vi "ws Spartan Event Log.vi"(4 "Force Archive? (f)":bool, 5 "error in (no error)":errorcluster, 6 "username (\"\")":string, 7 "module (\"\")":string, 8 "message (\"\")":string) -> (0 "error out":errorcluster)   [LabVIEW 2011]
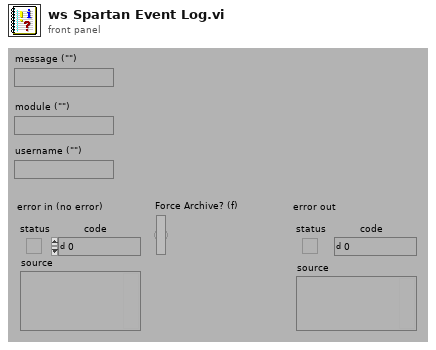
[diagram p1: front panel]
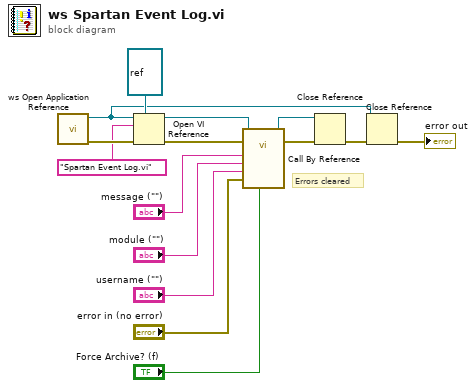
[diagram p0: block diagram]
diagram:
  # "Errors cleared"
  n1 = call "ws Open Application Reference.vi"() -> ("error out"=w15:errorcluster, "application reference"=w2:refnum<vi>)  [unwired: 10 in]
  n2 = Open VI Reference(type specifier VI Refnum (for type only)=refnum<vi> refnum, application reference (local)=w2, vi path="Spartan Event Log.vi", error in (no error)=w15) -> (vi reference=w11:refnum<vi>, error out=w13:errorcluster)  [unwired: 2 in]
  n3 = call-by-ref "?"(reference=w11, error in=w13, "Force Archive? (f)"="Force Archive? (f)", 5:"error in (no error)"="error in (no error)", "username (\"\")"="username (\"\")", "module (\"\")"="module (\"\")", "message (\"\")"="message (\"\")") -> (reference out=w5:refnum<vi>, error out=w4:errorcluster)  [unwired: 3 in, 1 out]
  n4 = Close Reference(reference=w5, error in (no error)=w4) -> (error out=w3:errorcluster)
  n5 = Close Reference(reference=w2, error in (no error)=w3) -> (error out=→"error out":errorcluster)
